vi "Generate Sequencer DVR.vi"(8 "Error In":errorcluster, 11 "Sequencer In":refnum<class "Sequencer.lvclass">) -> (0 "Error Out":errorcluster, 3 "Sequencer Out":refnum<class "Sequencer.lvclass">)   [LabVIEW 2019, in "Sequencer.lvclass"]
uses:
  Sequencer.lvclass
  Controls/Data.ctl
  Sequencer.lvclass/Sequencer.ctl
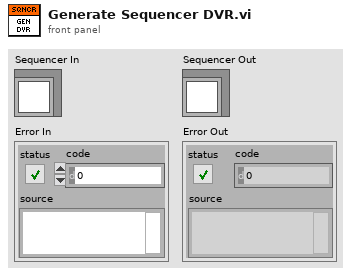
[diagram p1: front panel]
types:
  T1 = typedef "Sequencer.lvclass/Data.ctl" = cluster{"State":string}
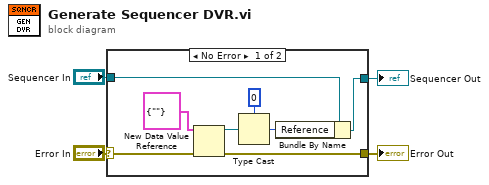
[diagram p0: block diagram]
diagram:
  n1 = case shown="No Error" "Error In" {
    selector: "Error In" -> [w12 w14]
    tunnel: "Sequencer In" -> [w9 w13]
    tunnel: [w8 w13] -> w3
    tunnel: [w7 w14] -> w1
    frame No Error {
      n2 = New Data Value Reference(data value=T1 {"State"=""} ("Data"), error in=w12) -> (data value reference=w11:refnum<data-value>, error out=w7:errorcluster)
      n3 = Type Cast(type=u64 0, x=w11) -> (*(type *) &x=w6:u64)
      n4 = Bundle By Name(cluster=w9, "Reference"=w6) -> (w8:refnum<class "Sequencer.lvclass">)
    }
    frame Error {
    }
  }
  "Error Out" <- w1
  "Sequencer Out" <- w3
